vi "Photocell.vi"(7 "Analog Ref Override":dbl, 8 "Error In":errorcluster, 10 "AI Channel":u8, 11 "LINX Resource":T1) -> (0 "Error Out":errorcluster, 2 "Value (0-100)":dbl, 3 "LINX Resource":T1)   [LabVIEW 2011, in "LVH-LINX.lvlib"]
uses:
  LVH-LINX.lvlib
  Private/Type Defs/LINX Ref.ctl
  Private/Type Defs/Platform.ctl
  Private/Type Defs/Interface.ctl
  Private/Device/Type Defs/LINX Device Config.ctl
  Private/Device/Type Defs/TCP Config.ctl
  Private/Type Defs/Device Family.ctl
  Private/Device/Device.lvlib
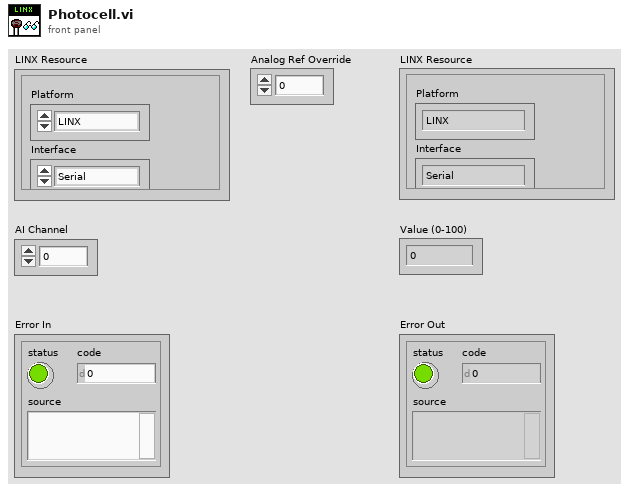
[diagram p1: front panel]
types:
  T1 = typedef "LVH-LINX.lvlib/LINX Ref.ctl" = cluster{"Platform":T2, "Interface":T3, "LINX Device Config":T4}
  T2 = typedef "LVH-LINX.lvlib/Platform.ctl" = enum16{"LINX", "myRIO"}
  T3 = typedef "LVH-LINX.lvlib/Interface.ctl" = enum16{"Serial", "TCP"}
  T4 = typedef "LVH-LINX.lvlib/Device.lvlib/LINX Device Config.ctl" = cluster{"Interface":T3, "COM Port":refnum<visa-resource-name>, "TCP Configuration":T5, "Device Family":T6, "Device ID":u8, "Device Name":string, "TCP Ref":refnum<k5>}
  T5 = typedef "LVH-LINX.lvlib/Device.lvlib/TCP Config.ctl" = cluster{"IP Address":string, "Port":u16}
  T6 = typedef "LVH-LINX.lvlib/Device Family.ctl" = enum8{"National Instruments", "Digilent", "Arduino"}
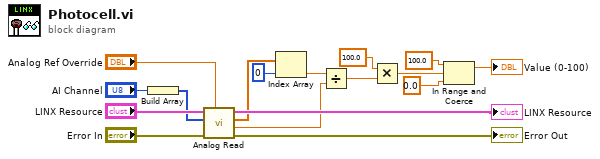
[diagram p0: block diagram]
diagram:
  n1 = Build Array("AI Channel") -> (w3:u8[])
  n2 = call "Analog Read.vi"("Analog Ref Override"="Analog Ref Override", "Error In"="Error In", "AI Channel(s)"=w3, "LINX Resource"="LINX Resource") -> ("Error Out"=→"Error Out":errorcluster, "AI Ref"=w1:dbl, "Voltages"=w6:dbl[], "LINX Resource"=→"LINX Resource":T1)  [unwired: 4 in]
  n3 = Index Array(array=w6, index=0) -> (element=w7:dbl)
  n4 = Divide(x=w7, y=w1) -> (x/y=w12:dbl)
  n5 = Multiply(x=100.0, y=w12) -> (x*y=w8:dbl)
  n6 = In Range and Coerce(upper limit=100.0, x=w8, lower limit=0.0) -> (coerced(x)=→"Value (0-100)":dbl)  [unwired: 1 out]
